vi "GenerateAbsolutleUnique2DArray.vi"(8 "Colums":i32=6, 11 "Rows":i32=3) -> (0 "2D Double Array":i32[][](array[numeric]), 2 "Table Control":string[][](table), 3 "2D String Array":string[][](array[string]))   [LabVIEW 2023]
uses:
  <vilib>/numeric/Random Number (Range) DBL.vi
  <vilib>/numeric/Random Number (Range) U64.vi
  <vilib>/numeric/sub_Random U32.vi
panel:
  out "Repeated attempt":i32
  out "?":i32
  out "?":i32
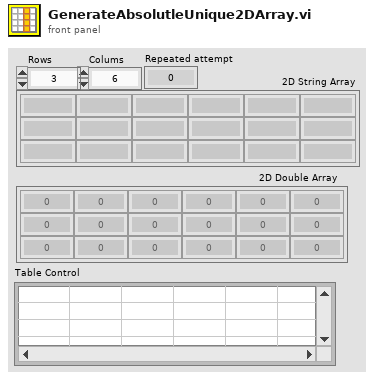
[diagram p1: front panel]
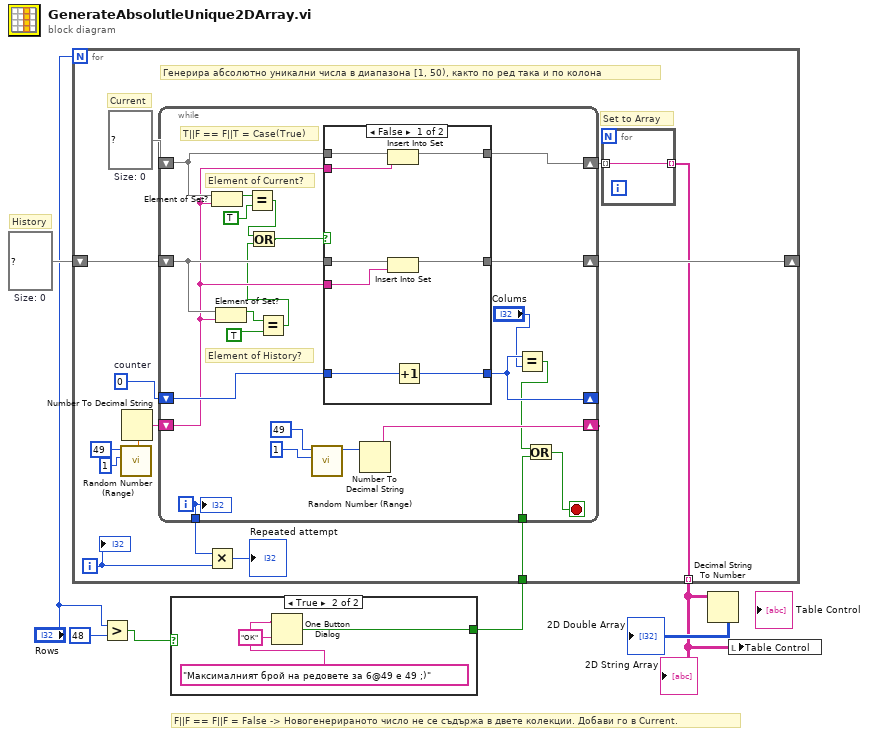
[diagram p0: block diagram]
diagram:
  w6 = set{string} {}  # Size: 0
  # "History"
  # "F||F == F||F = False -> Новогенерираното число не се съдържа в двете колекции. Добави го в Current."
  n1 = Greater?(x="Rows", y=48) -> (0:w3:bool)
  n2 = case shown="True" w3 {
    selector: w3 -> [w8 _]
    tunnel: [w8 w9] -> w2
    frame False {
    }
    frame True {
      n3 = One Button Dialog(message="Максималният брой на редовете за 6@49 е 49 ;)", button name ("OK")="ОК") -> (true=w9:bool)
    }
  }
  n4 = for {
    N: "Rows" -> [_]
    tunnel: [w12] -> w1 mode=indexing
    shift-right: [w18] -> _
    shift-left: w6 -> [w17]
    tunnel: w2 -> [w13]
    i -> [w15]
    w19 = set{string} {}  # Size: 0
    w21 = 0  # counter
    # "Current"
    # "Генерира абсолютно уникални числа в диапазона [1, 50), както по ред така и по колона"
    # "Set to Array"
    n5 = call-poly <vilib>:"Random Number (Range).vi"("lower bound (0)"=u64 1, "upper bound (100)"=u64 49) -> ("number"=w25:dbl)  [unwired: 9 in]
    n6 = Number To Decimal String(number=w25) -> (decimal integer string=w22:string)  [unwired: 1 in]
    n7 = while {
      shift-right: [w27] -> w20
      shift-left: w19 -> [w49]
      shift-right: [w42] -> _
      shift-left: w22 -> [w39]
      shift-right: [w47] -> _
      shift-left: w21 -> [w48]
      shift-right: [w41] -> w18
      shift-left: w17 -> [w40]
      tunnel: [w31] -> w16
      tunnel: w13 -> [w29]
      i -> [w31]
      stop <- w28 stop-if-true
      # "Element of Current?"
      # "Element of History?"
      # "T||F == F||T = Case(True)"
      n8 = Element of Set?(10:w39, 11:w49) -> (3:w36:bool)
      n9 = Element of Set?(10:w39, 11:w40) -> (3:w38:bool)
      n10 = Equal?(x=w36, y=TRUE) -> (x = y?=w33:bool)
      n11 = Equal?(x=w38, y=TRUE) -> (x = y?=w34:bool)
      n12 = Or(x=w33, y=w34) -> (x .or. y?=w32:bool)
      n13 = call-poly <vilib>:"Random Number (Range).vi"("lower bound (0)"=u64 1, "upper bound (100)"=u64 49) -> ("number"=w45:u64)  [unwired: 9 in]
      n14 = case shown="False" w32 {
        tunnel: w49 -> [w57 w60]
        tunnel: w39 -> [w51 _]
        tunnel: [w56 w60] -> w27
        tunnel: w48 -> [w54 w59]
        tunnel: [w55 w59] -> w47
        tunnel: [w52 w58] -> w41
        tunnel: w39 -> [w50 _]
        tunnel: w40 -> [w53 w58]
        frame False {
          n15 = Insert Into Set(10:w51, 11:w57) -> (3:w56:set{string})  [unwired: 1 out]
          n16 = Insert Into Set(10:w50, 11:w53) -> (3:w52:set{string})  [unwired: 1 out]
          n17 = Increment(x=w54) -> (x+1=w55:i32)
        }
        frame True {
        }
      }
      n18 = Number To Decimal String(number=w45) -> (decimal integer string=w42:string)  [unwired: 1 in]
      n19 = Equal?(x=w47, y="Colums") -> (x = y?=w30:bool)
      n20 = Or(x=w30, y=w29) -> (x .or. y?=w28:bool)
      "?" <- w31
    }
    n21 = Multiply(x=w16, y=w15) -> (x*y=→"Repeated attempt":i32)
    n22 = for {
      tunnel: [w26] -> w12 mode=indexing
      tunnel: w20 -> [w26] mode=indexing
    }
    "?" <- w15
  }
  "2D String Array" <- w1
  n23 = Decimal String To Number(string=w1) -> (number=→"2D Double Array":i32[][])  [unwired: 2 in, 1 out]
  n24 = local write "Table Control"(w1) -> ()
